vi "AI_one.vi"() -> ()   [LabVIEW 2019]
panel:
  in  "BaudRate":u32=115200
  in  "AITotalCh#":i16=8
  in  "AIChannel(0 ~ 7)":i16
  out "AI data (float)":sgl format="%.2f"
  out "return":i16
  in  "DCON_AI_Module":T1={"ComPort"=1, "Address"=1, "Slot"=1, "CheckSum"=0, "TimeOut"=1000}
  in  "stop":bool
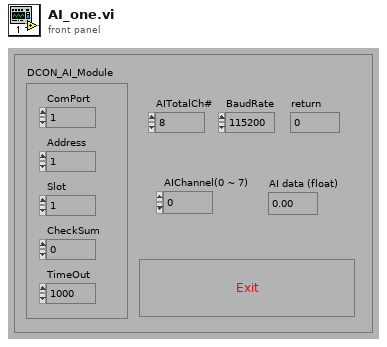
[diagram p1: front panel]
types:
  T1 = cluster{"ComPort":u8, "Address":i16, "Slot":i16, "CheckSum":i16, "TimeOut":i16}
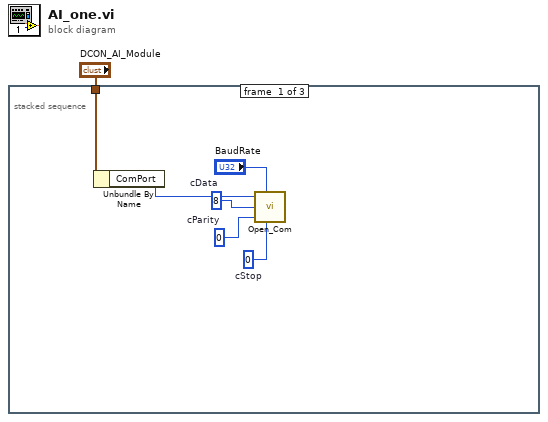
[diagram p0: block diagram]
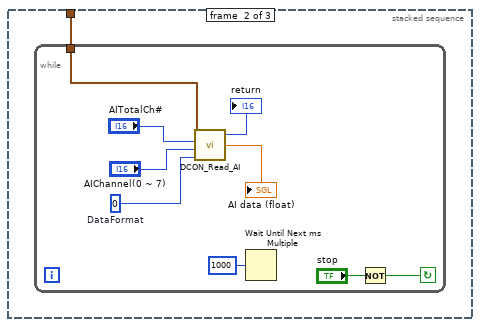
[diagram p2: hidden frame]
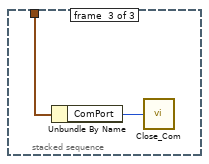
[diagram p3: hidden frame]
diagram:
  n1 = stacked-sequence {
    tunnel: "DCON_AI_Module" -> [w4 w8 w19]
    frame #0 {
      w5 = u8 0  # cStop
      w6 = u8 0  # cParity
      w7 = u8 8  # cData
      n2 = Unbundle By Name(w4) -> ("ComPort"=w3:u8)
      n3 = call "Open_Com.VI"("port number"=w3, "baudrate (115200)"="BaudRate", "data bit (8)"=w7, "parity (0: none)"=w6, "stop bit (0: 1 stop bit)"=w5) -> ()  [unwired: 1 out]
    }
    frame #1 {
      n4 = while {
        tunnel: w8 -> [w12]
        stop <- w17 continue-if-true
        w11 = i16 0  # DataFormat
        n5 = call "DCON_Read_AI.vi"("DataFormat (0)"=w11, "AIChannel"="AIChannel(0 ~ 7)", "AITotalCh"="AITotalCh#", "DCON_Module"=w12) -> ("Float_AI"=→"AI data (float)":sgl, "return"=→"return":i16)  [unwired: 1 out]
        n6 = Wait Until Next ms Multiple(millisecond multiple=u32 1000) -> ()  [unwired: 1 out]
        n7 = Not(x="stop") -> (.not. x?=w17:bool)
      }
    }
    frame #2 {
      n8 = Unbundle By Name(w19) -> ("ComPort"=w18:u8)
      n9 = call "Close_Com.vi"("port number"=w18) -> ()  [unwired: 1 out]
    }
  }
